vi "3DpictureObjectRemove.vi"() -> ()   [LabVIEW 2021]
uses:
  <vilib>/picture/3D Picture Control/Object/Create Object (name).vi
  <vilib>/picture/3D Picture Control/Object/Create Object (drawable).vi
  <vilib>/picture/3D Picture Control/Object/Add Object (no reference).vi
  <vilib>/picture/3D Picture Control/Object/Add Object (reference).vi
  <vilib>/picture/3D Picture Control/NI_3D Picture Control.lvlib
  <vilib>/picture/3D Picture Control/Object/Create Object (drawable with reference).vi
panel:
  in  "removeBoxByRef":bool
  in  "removeBoxByName":bool
  in  "Stop":bool
  in  "addBox":bool
  out "3D Picture":refnum<vi>(3d-picture)
  # "For some reason they don't expose the \"Remove\" method through a VI like the \"Add\".."
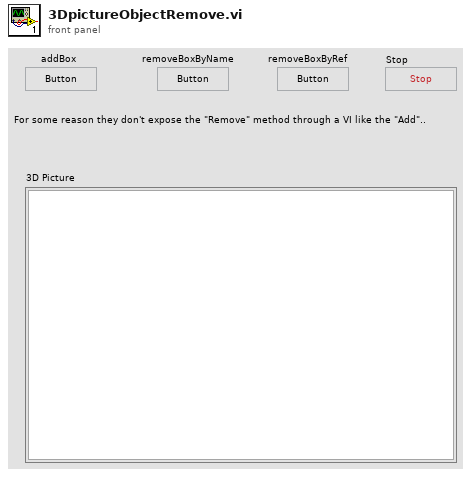
[diagram p1: front panel]
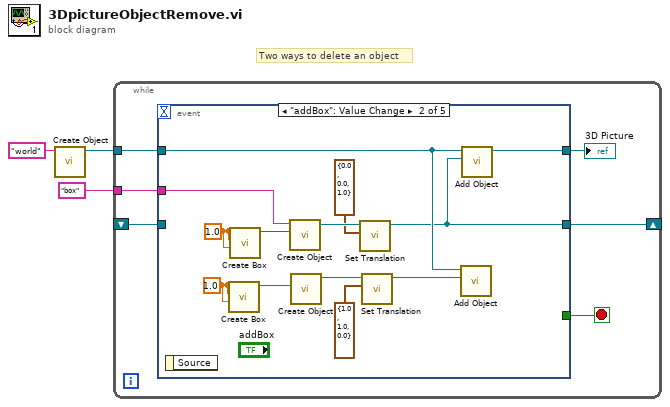
[diagram p0: block diagram]
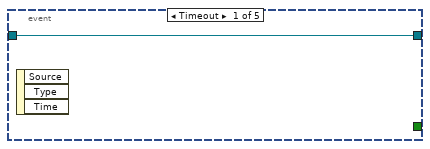
[diagram p2: hidden frame]
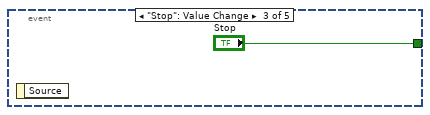
[diagram p3: hidden frame]
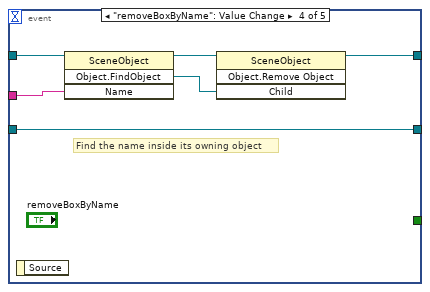
[diagram p4: hidden frame]
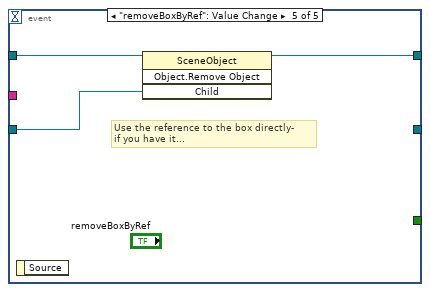
[diagram p5: hidden frame]
diagram:
  # "Two ways to delete an object"
  n1 = call-poly <vilib>:"Create Object.vi"("Name"="world") -> ("Scene:New Object"=w3:refnum<vi>)  [unwired: 9 in, 1 out]
  n2 = while {
    tunnel: w3 -> [w9]
    tunnel: "box" ("Name") -> [w6]
    shift-right: [w5] -> _
    shift-left: _ -> [w4]
    stop <- w7 stop-if-true
    n3 = event shown="[1] \"addBox\": Value Change" {
      selector: _ -> [_ _ _ _ _]
      dyn-events: _ -> [_ _ _ _ _]
      timeout: _ -> [_ _ _ _ _]
      tunnel: w9 -> [_ w14 _ w30 w32]
      tunnel: [_ w22 _ w26 w31] -> w8
      tunnel: [_ _ "Stop" _ _] -> w7
      tunnel: w6 -> [_ w21 _ w28 _]
      tunnel: [w10 w13 _ w25 _] -> w5
      tunnel: w4 -> [w10 _ _ w25 w33]
      event Timeout {
        n4 = event-data() -> ()  [unwired: 1 in, 3 out]
      }
      event "addBox": Value Change {
        w18 = sgl 1.0 ("Length X")
        w23 = sgl 1.0 ("Length X")
        n5 = event-data() -> ()  [unwired: 1 in, 1 out]
        n6 = call <vilib>:"Create Box.vi"("Length Z"=w18, "Length Y"=w18, "Length X"=w18) -> ("New Box Refnum"=w11:refnum<vi>)  [unwired: 7 in, 1 out]
        n7 = call <vilib>:"Create Box.vi"("Length Z"=w23, "Length Y"=w23, "Length X"=w23) -> ("New Box Refnum"=w12:refnum<vi>)  [unwired: 7 in, 1 out]
        n8 = call-poly <vilib>:"Create Object.vi"("Geometry or text"=w12, "Name"=w21) -> ("Scene:New Object"=w17:refnum<vi>)  [unwired: 7 in, 2 out]
        n9 = call-poly <vilib>:"Create Object.vi"("Geometry"=w11) -> ("Scene:New Object"=w20:refnum<vi>)  [unwired: 9 in, 1 out]
        n10 = call <vilib>:"Set Translation.vi"("Translation"=cluster{"X":sgl, "Y":sgl, "Z":sgl} {"X"=0.0, "Y"=0.0, "Z"=1.0}, "Scene Object"=w17) -> ("Translated Object"=w13:refnum<vi>)  [unwired: 8 in, 1 out]
        n11 = call <vilib>:"Set Translation.vi"("Translation"=cluster{"X":sgl, "Y":sgl, "Z":sgl} {"X"=1.0, "Y"=1.0, "Z"=0.0}, "Scene Object"=w20) -> ("Translated Object"=w15:refnum<vi>)  [unwired: 8 in, 1 out]
        n12 = call-poly <vilib>:"Add Object.vi"("New Object In"=w15, "Scene Object In"=w14) -> ()  [unwired: 8 in, 2 out]
        n13 = call-poly <vilib>:"Add Object.vi"("New Object In"=w13, "Scene Object In"=w14) -> ("Scene Object Out"=w22:refnum<vi>)  [unwired: 7 in, 2 out]
      }
      event "Stop": Value Change {
        n14 = event-data() -> ()  [unwired: 1 in, 1 out]
      }
      event "removeBoxByName": Value Change {
        # "Find the name inside its owning object"
        n15 = event-data() -> ()  [unwired: 1 in, 1 out]
        n16 = invoke class="SceneObject" method="Object.FindObject"(reference=w30, "Name"=w28) -> (reference out=w29:refnum<vi>, "FindObject"=w27:refnum<vi>)  [unwired: 2 in, 2 out]
        n17 = invoke class="SceneObject" method="Object.Remove Object"(reference=w29, "Child"=w27) -> (reference out=w26:refnum<vi>)  [unwired: 2 in, 3 out]
      }
      event "removeBoxByRef": Value Change {
        # "Use the reference to the box directly- \nif you have it..."
        n18 = event-data() -> ()  [unwired: 1 in, 1 out]
        n19 = invoke class="SceneObject" method="Object.Remove Object"(reference=w32, "Child"=w33) -> (reference out=w31:refnum<vi>)  [unwired: 2 in, 3 out]
      }
    }
    "3D Picture" <- w8
  }
